vi "Read Module Reference.vi"(8 "error in":errorcluster, 11 "execution unit":refnum<class "Execution Unit.lvclass">) -> (0 "error out":errorcluster, 2 "module reference":T1, 3 "execution unit out":refnum<class "Execution Unit.lvclass">)   [LabVIEW 2020, in "AIM MIL-STD-1553 Engine.lvlib" / "Implementation.lvlib" / "Execution Unit.lvclass"]
uses:
  Execution Unit.lvclass
  Hardware API/Module Reference.ctl
  Execution Unit.lvclass/Execution Unit.ctl
  Hardware API/AIM MIL-STD-1553 Hardware API.lvlib
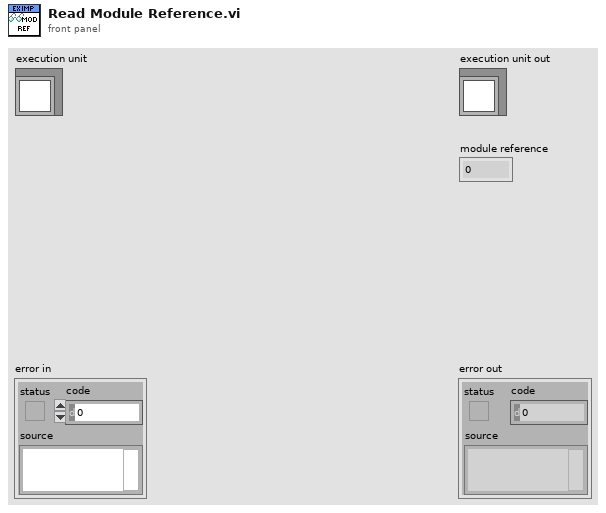
[diagram p1: front panel]
types:
  T1 = typedef "AIM MIL-STD-1553 Hardware API.lvlib/Module Reference.ctl" = u32
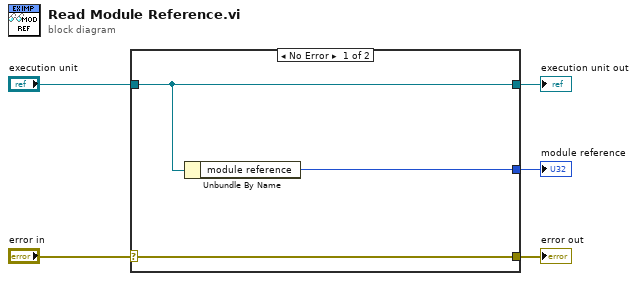
[diagram p0: block diagram]
diagram:
  n1 = case shown="No Error" "error in" {
    selector: "error in" -> [w8 w9]
    tunnel: [w8 w9] -> w4
    tunnel: [w7 w10] -> w2
    tunnel: "execution unit" -> [w7 w10]
    tunnel: [w6 _] -> w1
    frame No Error {
      n2 = Unbundle By Name(w7) -> ("module reference"=w6:T1)
    }
    frame Error {
    }
  }
  "error out" <- w4
  "execution unit out" <- w2
  "module reference" <- w1
